vi "Close Module.vi"(8 "error in (no error)":errorcluster, 9 "Wait for stop?":bool, 11 "Module Admin in":refnum<class "Delacor_lib_QMH_Cloneable Module Admin.lvclass">) -> (0 "error out":errorcluster, 1 "External Launch":bool, 3 "Module Admin out":refnum<class "Delacor_lib_QMH_Cloneable Module Admin.lvclass">)   [LabVIEW 2018, in "Timer Module.lvlib"]
doc: "Destroy the Broadcast Events and Request Events (if this was the first instance). Reset flags stored in Module Admin class.\n_____\nBased on Delacor QMH Project Template 4.1.0.56."
uses:
  Timer Module.lvlib
  <vilib>/Delacor/Delacor QMH/Libraries/Cloneable Module Admin_class/Delacor_lib_QMH_Cloneable Module Admin.lvclass
  C:/Program Files (x86)/National Instruments/LabVIEW 2018/vi.lib/Delacor/Delacor QMH/Libraries/Module Admin_class/Delacor_lib_QMH_Module Admin.lvclass
  <vilib>/Delacor/Delacor QMH/Libraries/Cloneable Module Admin_class/Delacor_lib_QMH_Cloneable Module Admin.lvclass/Delacor_lib_QMH_Cloneable Module Admin.ctl
  <vilib>/Delacor/Delacor QMH/Libraries/Module Admin_class/Delacor_lib_QMH_Module Admin.lvclass/Delacor_lib_QMH_Module Admin.ctl
  <vilib>/Delacor/Delacor QMH/Libraries/Cloneable Module Admin_class/Delacor_lib_QMH_Get First.vi
  <vilib>/Delacor/Delacor QMH/Libraries/Cloneable Module Admin_class/Delacor_lib_QMH_Get Module ID.vi
  <vilib>/Delacor/Delacor QMH/Libraries/Module Admin_class/Delacor_lib_QMH_Get External Launch.vi
  Clone Registration/Clone Registration.lvlib
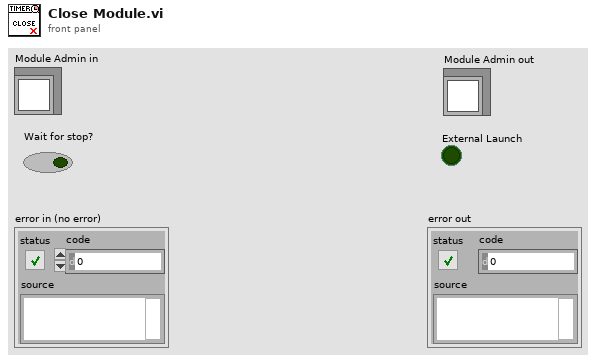
[diagram p1: front panel]
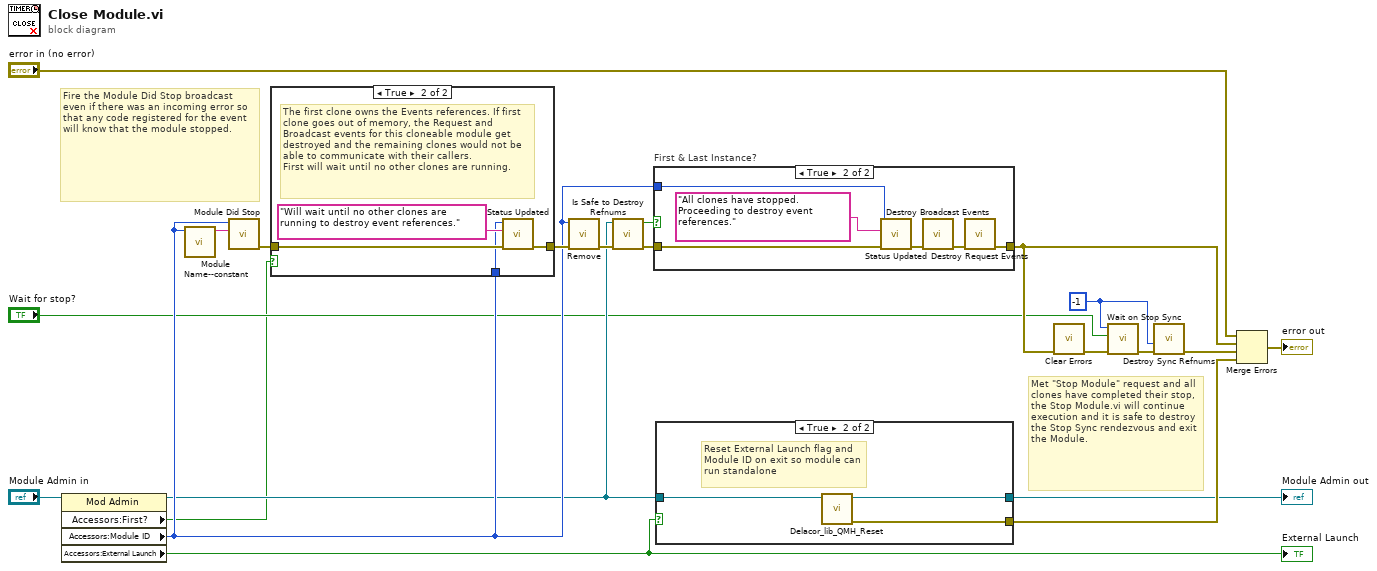
[diagram p0: block diagram]
diagram:
  w7 = -1 ("Module ID")
  # "Fire the Module Did Stop broadcast even if there was an incoming error so that any code registered for the event will know that the module stopped."
  # "Met \"Stop Module\" request and all clones have completed their stop, the Stop Module.vi will continue execution and it is safe to destroy the Stop Sync rendezvous and exit the Module."
  n1 = property class="Mod Admin"(reference="Module Admin in") -> (reference out=w16:refnum<class "Delacor_lib_QMH_Cloneable Module Admin.lvclass">, "Accessors:First?"=w4:bool, "Accessors:Module ID"=w20:i32, "Accessors:External Launch"=w3:bool)  [unwired: 1 in, 1 out]
  "External Launch" <- w3
  n2 = call "Module Name--constant.vi"("Module ID"=w20) -> ("Module Name"=w2:string)  [unwired: 10 in]
  n3 = call "Module Did Stop.vi"("Origin"=w2, "Module ID"=w20) -> ("error out"=w11:errorcluster)  [unwired: 9 in]
  n4 = case shown="True" w4 {
    tunnel: w11 -> [w22 w26]
    tunnel: w20 -> [_ w24]
    tunnel: [w22 w23] -> w21
    frame False {
    }
    frame True {
      # "The first clone owns the Events references. If first clone goes out of memory, the Request and Broadcast events for this cloneable module get destroyed and the remaining clones would not be able to communicate with their callers.\nFirst will wait until no other clones are running."
      n5 = call "Status Updated.vi"("error in (no error)"=w26, "Status"="Will wait until no other clones are running to destroy event references." ("format string"), "Module ID"=w24) -> ("error out"=w23:errorcluster)  [unwired: 8 in]
    }
  }
  n6 = call "Remove.vi"("error in (no error)"=w21, "Module ID"=w20) -> ("error out"=w17:errorcluster)  [unwired: 8 in, 1 out]
  n7 = call "Is Safe to Destroy Refnums.vi"("error in (no error)"=w17, "Module Admin"=w16) -> ("error out"=w13:errorcluster, "Destroy Broadcast & Request Event Refs?"=w14:bool)  [unwired: 8 in]
  n8 = case "First & Last Instance?" shown="True" w14 {
    tunnel: w13 -> [w27 w31]
    tunnel: [w27 w33] -> w19
    tunnel: w20 -> [_ w29]
    frame False {
    }
    frame True {
      n9 = call "Status Updated.vi"("error in (no error)"=w31, "Status"="All clones have stopped. Proceeding to destroy event references.", "Module ID"=w29) -> ("error out"=w30:errorcluster)  [unwired: 8 in]
      n10 = call "Destroy Broadcast Events.vi"("error in (no error)"=w30) -> ("error out"=w32:errorcluster)  [unwired: 10 in]
      n11 = call "Destroy Request Events.vi"("error in (no error)"=w32) -> ("error out"=w33:errorcluster)  [unwired: 10 in]
    }
  }
  n12 = case shown="True" w3 {
    tunnel: w16 -> [w34 w37]
    tunnel: [w34 w36] -> w12
    tunnel: [_ w35] -> w18
    frame False {
    }
    frame True {
      # "Reset External Launch flag and Module ID on exit so module can run standalone"
      n13 = call-dynamic "Delacor_lib_QMH_Reset.vi"("Mod Admin in"=w37) -> ("error out"=w35:errorcluster, "Mod Admin out"=w36:refnum<class "Delacor_lib_QMH_Cloneable Module Admin.lvclass">)  [unwired: 9 in]
    }
  }
  "Module Admin out" <- w12
  n14 = call <vilib>:"Clear Errors.vi"("error in (no error)"=w19) -> ("error out"=w6:errorcluster)  [unwired: 5 in, 1 out]
  n15 = call "Wait on Stop Sync.vi"("error in (no error)"=w6, "Wait for Module to stop?"="Wait for stop?", "Module ID"=w7) -> ("error out"=w10:errorcluster)  [unwired: 8 in]
  n16 = call "Destroy Sync Refnums.vi"("error in (no error)"=w10, "Module ID"=w7) -> ("error out"=w8:errorcluster)  [unwired: 9 in]
  n17 = Merge Errors("error in (no error)", w19, w8, w18) -> (→"error out":errorcluster)
